vi "Matlab_2.vi"(0 "additonal Mass[g]":dbl, 1 "Subject ID":dbl, 2 "Impactor ID":dbl, 3 "comment":string, 5 "loginName":string, 7 "Impact Speed":dbl, 9 "Pendel Velocity":dbl, 11 "Fehler (Eingang, kein Fehler)":errorcluster, 12 "Humidity":dbl) -> (4 "Exp_id":i32, 15 "Fehler (Ausgang)":errorcluster)   [LabVIEW 2020]
panel:
  out "DB error":bool
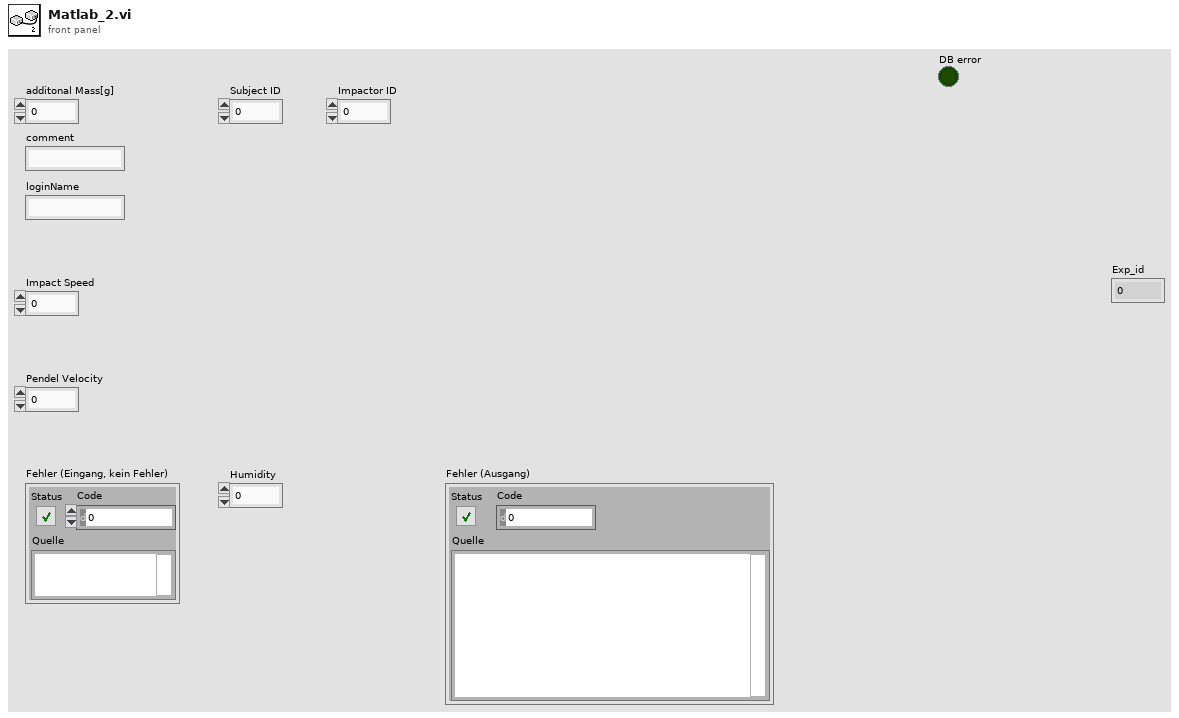
[diagram p1: front panel]
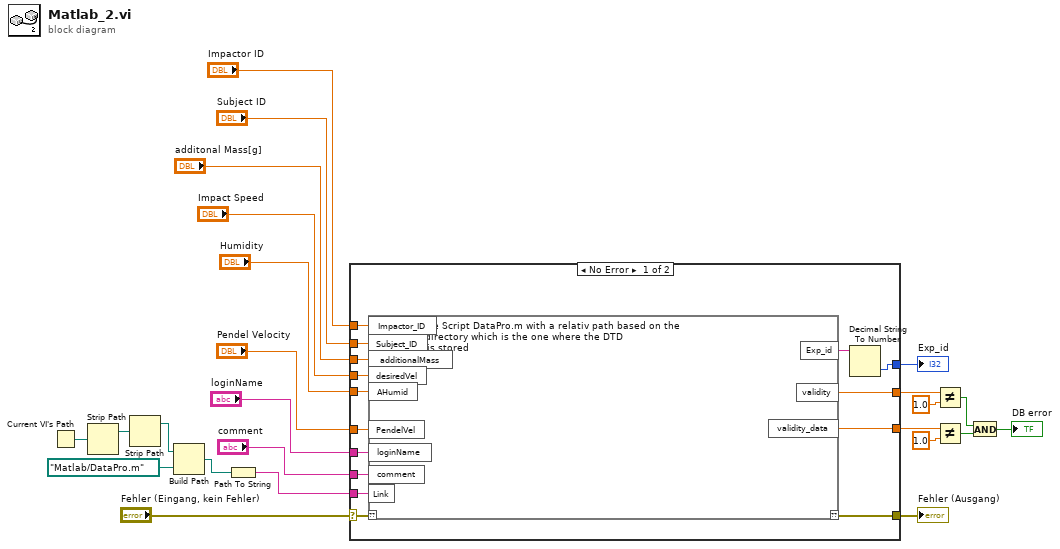
[diagram p0: block diagram]
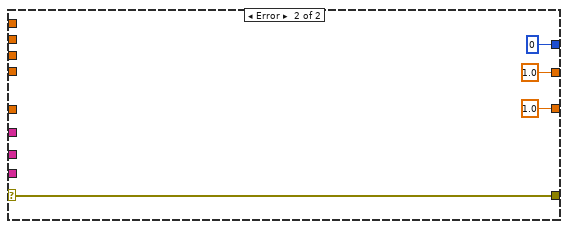
[diagram p2: hidden frame]
diagram:
  n1 = Current VI's Path() -> (path=w13:path)
  n2 = Strip Path(path=w13) -> (stripped path=w12:path)  [unwired: 1 out]
  n3 = Strip Path(path=w12) -> (stripped path=w11:path)  [unwired: 1 out]
  n4 = Build Path(base path=w11, name or relative path=path "Matlab/DataPro.m" ("Name oder relativer Pfad")) -> (appended path=w9:path)
  n5 = Path To String(path=w9) -> (string=w8:string)
  n6 = case shown="No Error" "Fehler (Eingang, kein Fehler)" {
    selector: "Fehler (Eingang, kein Fehler)" -> [w28 w42]
    tunnel: [w39 1.0] -> w24
    tunnel: "loginName" -> [w38 _]
    tunnel: "Impact Speed" -> [w37 _]
    tunnel: "Pendel Velocity" -> [w36 _]
    tunnel: "additonal Mass[g]" -> [w35 _]
    tunnel: "Humidity" -> [w34 _]
    tunnel: "Subject ID" -> [w33 _]
    tunnel: "Impactor ID" -> [w32 _]
    tunnel: [w31 w42] -> w15
    tunnel: "comment" -> [w30 _]
    tunnel: w8 -> [w29 _]
    tunnel: [w27 1.0] -> w5
    tunnel: [w25 0] -> w1
    frame No Error {
      n7 = script code="%Calling the Script DataPro.m with a relativ path based on the \n%current directory which is the one where the DTD \n% project is stored\nrun(Link)"("??"=w28, "Impactor_ID"=w32, "Subject_ID"=w33, "additionalMass"=w35, "desiredVel"=w37, "AHumid"=w34, "PendelVel"=w36, "loginName"=w38, "comment"=w30, "Link"=w29) -> ("??"=w31:errorcluster, "validity_data"=w39:dbl, "validity"=w27:dbl, "Exp_id"=w26:string)
      n8 = Decimal String To Number(string=w26) -> (number=w25:i32)  [unwired: 2 in, 1 out]
    }
    frame Error {
    }
  }
  "Fehler (Ausgang)" <- w15
  "Exp_id" <- w1
  n9 = Not Equal?(x=w5, y=1.0) -> (x != y?=w4:bool)
  n10 = Not Equal?(x=w24, y=1.0) -> (x != y?=w3:bool)
  n11 = And(x=w4, y=w3) -> (x .and. y?=→"DB error":bool)
